vi "FlatToRichniswitch_grpc_ConnectMultipleResponse.vi"(5 "OutputClusterType":T1, 11 "InputCluster":T2) -> (3 "OutputCluster":T1)   [LabVIEW 2021, in "NI Switch_client.lvlib"]
uses:
  NI Switch_client.lvlib
  niswitch_grpc_ConnectMultipleResponse_Flat.ctl
  niswitch_grpc_ConnectMultipleResponse.ctl
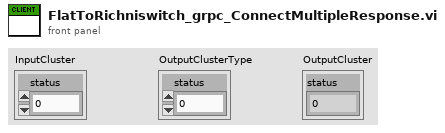
[diagram p1: front panel]
types:
  T1 = typedef "NI Switch_client.lvlib/niswitch_grpc_ConnectMultipleResponse.ctl" = cluster{"status":i32}
  T2 = typedef "NI Switch_client.lvlib/niswitch_grpc_ConnectMultipleResponse_Flat.ctl" = cluster{"status":i32}
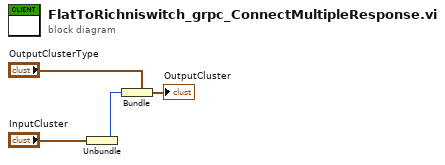
[diagram p0: block diagram]
diagram:
  n1 = Unbundle "Unbundle"("InputCluster") -> ("status"=w1:i32)
  n2 = Bundle "Bundle"(cluster="OutputClusterType", "status"=w1) -> (→"OutputCluster":T1)
